vi "FitGaussian2D.vi"() -> ()   [LabVIEW 2009]
panel:
  in  "Data":dbl[][](graph)
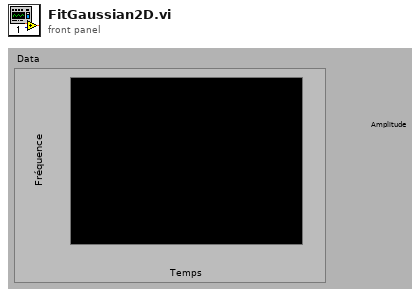
[diagram p1: front panel]
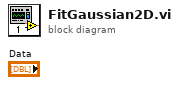
[diagram p0: block diagram]
diagram:
